vi "CLSUIP_RetoolVI.vi"(8 "error in (no error)":errorcluster, 11 "VIRetooler":refnum<class "VIRetooler.lvclass">) -> (0 "error out":errorcluster, 1 "NewItemID":string, 3 "VIRetooler out":refnum<class "VIRetooler.lvclass">)   [LabVIEW 2021, in "MemberVICreation.lvlib" / "VIRetooler.lvclass"]
uses:
  <resource>/Framework/Providers/LVClassLibrary/NewAccessors/VIRetooler/VIRetooler.lvclass
  <resource>/Framework/Providers/LVClassLibrary/NewAccessors/VIRetooler/CLSUIP_OverrideErrMsgs.vi
  <resource>/Framework/Providers/LVClassLibrary/NewAccessors/MemberVICreation.lvlib
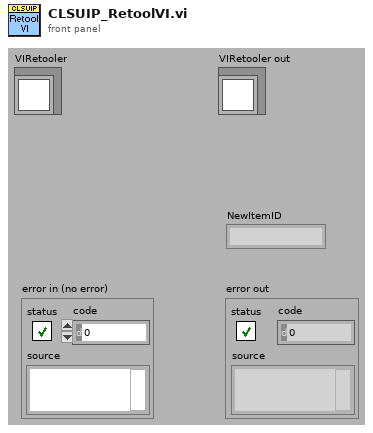
[diagram p1: front panel]
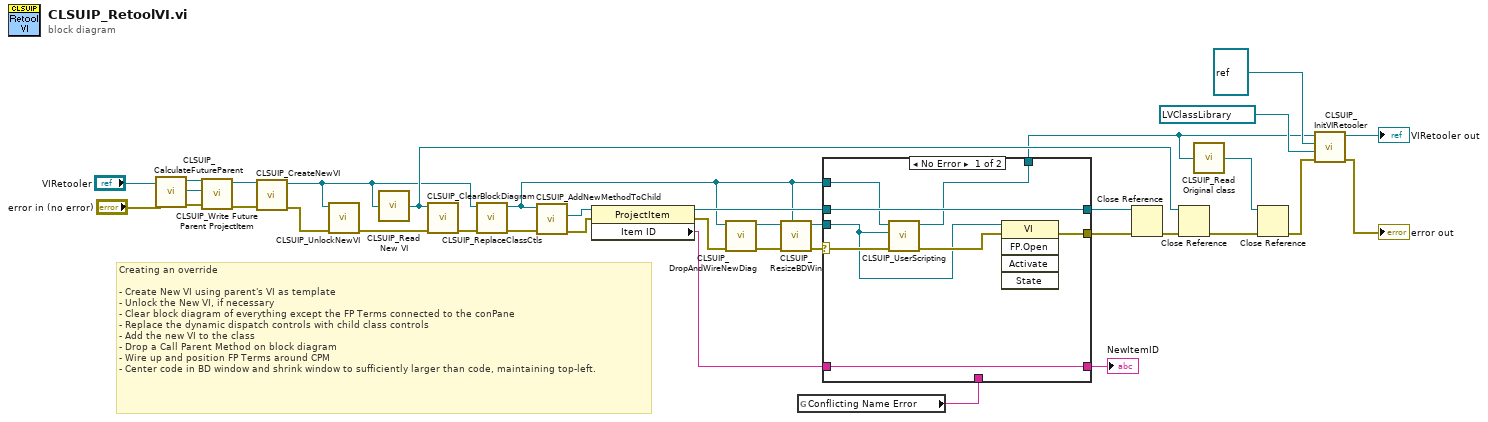
[diagram p0: block diagram]
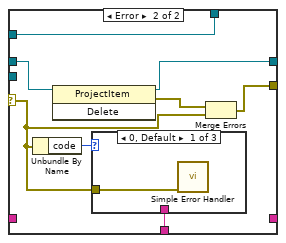
[diagram p2: hidden frame]
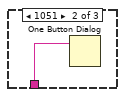
[diagram p3: hidden frame]
diagram:
  # "Creating an override\n\n- Create New VI using parent's VI as template\n- Unlock the New VI, if necessary\n- Clear block diagram of everything except the FP Terms connected to the conPane\n- Replace the dynamic dispatch controls with child class controls\n- Add the new VI to the class\n- Drop a Call Parent Method on block diagram\n- Wire up and position FP Terms around CPM\n- Center code in BD window and shrink window to sufficiently larger than code, maintaining top-left."
  n1 = call <resource>:"CLSUIP_CalculateFutureParent.vi"("error in (no error)"="error in (no error)", "VIRetooler in"="VIRetooler") -> ("error out"=w5:errorcluster, "NewParentItem"=w4:refnum<vi>, "VIRetooler out"=w3:refnum<class "VIRetooler.lvclass">)  [unwired: 7 in]
  n2 = call-dynamic "CLSUIP_Write Future Parent ProjectItem.vi"("error in (no error)"=w5, "Future Parent ProjectItem"=w4, "VIRetooler in"=w3) -> ("error out"=w1:errorcluster, "VIRetooler out"=w2:refnum<class "VIRetooler.lvclass">)  [unwired: 7 in]
  n3 = call <resource>:"CLSUIP_CreateNewVI.vi"("VIRetooler"=w2, "error in (no error)"=w1) -> ("VIRetooler out"=w18:refnum<class "VIRetooler.lvclass">, "error out"=w27:errorcluster)  [unwired: 6 out]
  n4 = call <resource>:"CLSUIP_UnlockNewVI.vi"("error in (no error)"=w27, "VIRetooler"=w18) -> ("error out"=w26:errorcluster)  [unwired: 1 in, 8 out]
  n5 = call <resource>:"CLSUIP_Read New VI.vi"("VIRetooler.lvclass in"=w18) -> ("New VI"=w23:refnum<vi>)
  n6 = call <resource>:"CLSUIP_ClearBlockDiagram.vi"("error in (no error)"=w26, "VI Refnum"=w23) -> ("error out"=w36:errorcluster)  [unwired: 9 out]
  n7 = call <resource>:"CLSUIP_ReplaceClassCtls.vi"("error in (no error)"=w36, "VIRetooler"=w18) -> ("error out"=w35:errorcluster, "VIRetooler out"=w9:refnum<class "VIRetooler.lvclass">)  [unwired: 2 in, 2 out]
  n8 = call <resource>:"CLSUIP_AddNewMethodToChild.vi"("error in (no error)"=w35, "VIRetooler"=w9) -> ("error out"=w33:errorcluster, "AddItemFromMemory"=w34:refnum<vi>)  [unwired: 1 in, 4 out]
  n9 = property on="Property Node" class="ProjectItem"(reference=w34, error in=w33) -> (reference out=w28:refnum<vi>, error out=w32:errorcluster, "Item ID"=w29:string)
  n10 = call-dynamic "CLSUIP_DropAndWireNewDiag.vi"("error in (no error)"=w32, "VIRetooler"=w9) -> ("error out"=w12:errorcluster, "VI Refnum out"=w11:refnum<vi>)  [unwired: 4 out]
  n11 = call-dynamic "CLSUIP_ResizeBDWin.vi"("VIRetooler in"=w9, "error in (no error)"=w12, "VI Refnum"=w11) -> ("error out"=w13:errorcluster, "VI Refnum out"=w10:refnum<vi>)  [unwired: 1 in, 6 out]
  n12 = global read "CLSUIP_OverrideErrMsgs.vi" "Conflicting Name Error"() -> (w31:string)
  n13 = case shown="No Error" w13 {
    selector: w13 -> [w41 w50]
    tunnel: w10 -> [w37 _]
    tunnel: [w44 w51] -> w24
    tunnel: w31 -> [_ w49]
    tunnel: [w43 _] -> w30
    tunnel: w29 -> [w43 _]
    tunnel: w28 -> [w42 w48]
    tunnel: [w42 w47] -> w22
    tunnel: w9 -> [w39 w45]
    tunnel: [w38 w45] -> w8
    frame No Error {
      n14 = call-dynamic "CLSUIP_UserScripting.vi"("error in"=w41, "VI Refnum in"=w37, "VIRetooler"=w39) -> ("error out"=w40:errorcluster, "VIRetooler out"=w38:refnum<class "VIRetooler.lvclass">)  [unwired: 7 in]
      n15 = invoke on="Invoke Node" class="VI" method="FP.Open"(reference=w37, error in=w40) -> (error out=w44:errorcluster)  [unwired: 3 in, 4 out]
    }
    frame Error {
      n16 = Unbundle By Name(w50) -> ("code"=w46:i32)
      n17 = invoke on="Invoke Node" class="ProjectItem" method="Delete"(reference=w48) -> (reference out=w47:refnum<vi>, error out=w52:errorcluster)  [unwired: 2 in, 1 out]
      n18 = case shown="0, Default" w46 {
        tunnel: w50 -> [w53 _ _]
        tunnel: w49 -> [_ w54 _]
        frame 0, Default {
          n19 = call <vilib>:"Simple Error Handler.vi"("error in (no error)"=w53) -> ()  [unwired: 1 in, 8 out]
        }
        frame 1051 {
          n20 = One Button Dialog(message=w54) -> ()  [unwired: 2 out]
        }
        frame 1040 {
          # "This case is because they cancelled the password prompt. It doesn't need further handling."
        }
      }
      n21 = Merge Errors(w52, w50) -> (w51:errorcluster)
    }
  }
  "NewItemID" <- w30
  n22 = Close Reference(reference=w22, error in (no error)=w24) -> (error out=w25:errorcluster)
  n23 = Close Reference(reference=w23, error in (no error)=w25) -> (error out=w16:errorcluster)
  n24 = call <resource>:"CLSUIP_Read Original class.vi"("VIRetooler.lvclass in"=w8) -> ("Orig class"=w15:refnum<vi>)
  n25 = Close Reference(reference=w15, error in (no error)=w16) -> (error out=w14:errorcluster)
  n26 = call <resource>:"CLSUIP_InitVIRetooler.vi"("error in (no error)"=w14, "Replacement class"=refnum<vi> refnum, "Member VI"=refnum<vi> refnum, "VIRetooler in"=w8) -> ("error out"=→"error out":errorcluster, "VIRetooler out"=→"VIRetooler out":refnum<class "VIRetooler.lvclass">)  [unwired: 6 out]
